vi "Set Password Display.vi"(8 "error in (no error)":errorcluster, 10 "Password Display":bool, 11 "Filled Text Fields in":refnum<class "Filled Text Fields.lvclass">) -> (0 "error out":errorcluster, 3 "Filled Text Fields out":refnum<class "Filled Text Fields.lvclass">)   [LabVIEW 2017, in "Filled Text Fields.lvlib" / "Filled Text Fields.lvclass"]
uses:
  Filled Text Fields.lvclass
  Filled Text Fields.lvclass/Filled Text Fields.ctl
  Filled Text Fields Actor Messages/onDisplayStateChange Msg/onDisplayStateChange Msg.lvclass
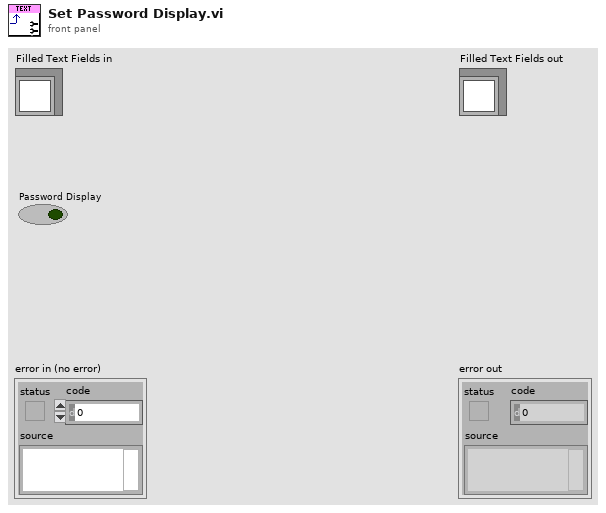
[diagram p1: front panel]
types:
  T1 = typedef "Theme.lvlib/Theme.Font.lvclass/Font.ctl" = cluster{"Size":u32, "Shrink Size":u32, "Name":string, "Password Display":bool}
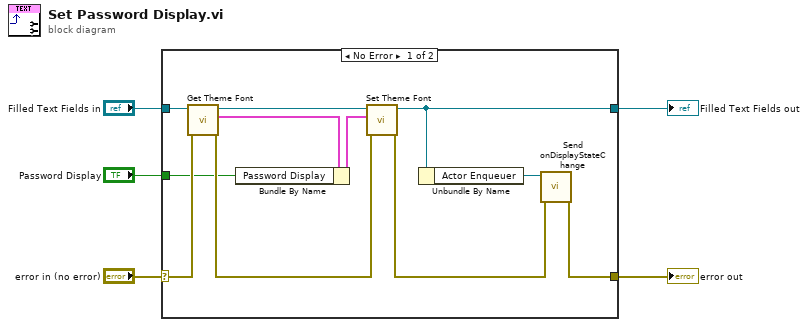
[diagram p0: block diagram]
diagram:
  n1 = case shown="No Error" "error in (no error)" {
    selector: "error in (no error)" -> [w10 w18]
    tunnel: [w15 w18] -> w4
    tunnel: [w12 w17] -> w2
    tunnel: "Filled Text Fields in" -> [w14 w17]
    tunnel: "Password Display" -> [w6 _]
    frame No Error {
      n2 = call "Get Theme Font.vi"("error in (no error)"=w10, "Filled Text Fields in"=w14) -> ("error out"=w9:errorcluster, "Properties:Font"=w11:T1, "Filled Text Fields out"=w13:refnum<class "Filled Text Fields.lvclass">)  [unwired: 7 in]
      n3 = Bundle By Name(cluster=w11, "Password Display"=w6) -> (w7:T1)
      n4 = call "Set Theme Font.vi"("error in (no error)"=w9, "Properties:Font"=w7, "Filled Text Fields in"=w13) -> ("error out"=w8:errorcluster, "Filled Text Fields out"=w12:refnum<class "Filled Text Fields.lvclass">)  [unwired: 7 in]
      n5 = Unbundle By Name(w12) -> ("Actor Enqueuer"=w16:refnum<class "Message Enqueuer.lvclass">)
      n6 = call "Send onDisplayStateChange.vi"("error in (no error)"=w8, "Message Enqueuer in"=w16) -> ("error out"=w15:errorcluster)  [unwired: 8 in, 1 out]
    }
    frame Error {
    }
  }
  "error out" <- w4
  "Filled Text Fields out" <- w2
